vi "Read Sensors v4.vi"(6 "I/O Cluster":T1, 10 "Use Simulation Data?":bool) -> (0 "Vicon Logging Signal":dbl, 3 "Sensors":T19)   [LabVIEW 2018]
uses:
  Sensor Data.ctl
  Target IO Initialized Cluster.ctl
  <vilib>/myRIO/Instrument Drivers/Onboard IO/AI/typedefs/AI Reference.ctl
  <vilib>/myRIO/Common/Instrument Driver Framework/Utilities/typedefs/myRIO Generic Hardware Reference.ctl
  <vilib>/myRIO/Common/Instrument Driver Framework/Utilities/typedefs/Hardware Version Enum.ctl
  <vilib>/myRIO/Common/Instrument Driver Framework/Utilities/typedefs/myRIO v1.0 Reference.ctl
  <vilib>/myRIO/Common/Instrument Driver Framework/Utilities/typedefs/Generic FPGA Reference.ctl
  <vilib>/myRIO/Common/Instrument Driver Framework/myRIO v1.0/AI/typedefs/AI Channels List.ctl
  <vilib>/myRIO/Common/Instrument Driver Framework/myRIO v1.0/AI/typedefs/AI Channels Enum.ctl
  <vilib>/myRIO/Common/Instrument Driver Framework/Utilities/typedefs/Analog Scaling Constants List.ctl
  <vilib>/myRIO/Common/Instrument Driver Framework/Utilities/typedefs/Analog Scaling Constants.ctl
  <vilib>/myRIO/Instrument Drivers/Onboard IO/AO/typedefs/AO Reference.ctl
  <vilib>/myRIO/Common/Instrument Driver Framework/myRIO v1.0/AO/typedefs/AO Channels List.ctl
  <vilib>/myRIO/Common/Instrument Driver Framework/myRIO v1.0/AO/typedefs/AO Channels Enum.ctl
  <vilib>/myRIO/Instrument Drivers/Onboard IO/Encoder/typedefs/Encoder Reference.ctl
  <vilib>/myRIO/Common/Instrument Driver Framework/myRIO v1.0/Encoder/typedefs/Encoder Channels Enum.ctl
  <vilib>/myRIO/Instrument Drivers/Onboard IO/DIO/typedefs/DIO Reference.ctl
  <vilib>/myRIO/Common/Instrument Driver Framework/myRIO v1.0/DIO/typedefs/DIO Channels List.ctl
  <vilib>/myRIO/Common/Instrument Driver Framework/myRIO v1.0/DIO/typedefs/DIO Channels Enum.ctl
  <vilib>/myRIO/Instrument Drivers/Onboard IO/AI/AI.lvlib
  <vilib>/myRIO/Instrument Drivers/Onboard IO/AO/AO.lvlib
  <vilib>/myRIO/Instrument Drivers/Onboard IO/Encoder/Encoder.lvlib
  <vilib>/myRIO/Instrument Drivers/Onboard IO/DIO/DIO.lvlib
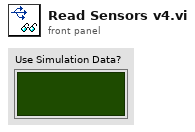
[diagram p1: front panel]
types:
  T1 = typedef "Target IO Initialized Cluster.ctl" = cluster{"AI Ref Out":T2, "AO Ref Out":T11, "Encoder Ref Out":T14, "UART resource name out":refnum<visa-resource-name>, "DIO Ref Out":T16}
  T2 = typedef "AI.lvlib/AI Reference.ctl" = cluster{"myRIO Reference":T3, "AI Channels List":T7, "AI Scaling Constants List":T9}
  T3 = typedef "myRIO Generic Hardware Reference.ctl" = cluster{"myRIO Model":T4, "myRIO Hardware Reference":T5}
  T4 = typedef "Hardware Version Enum.ctl" = enum16{"Unknown", "myRIO-1900", "myRIO-1950", "roboRIO", "NI ELVIS RIO CM", "ELVIS III"}
  T5 = typedef "myRIO v1.0 Reference.ctl" = cluster{"Generic FPGA Reference":T6, "Allow multiple opens":bool}
  T6 = typedef "Generic FPGA Reference.ctl" = refnum<k20>
  T7 = typedef "AI Channels List.ctl" = T8[]
  T8 = typedef "AI Channels Enum.ctl" = enum16{"Not Connected", "AudioIn/Left", "AudioIn/Right", "C/AI0", "C/AI1", "A/AI0", "A/AI1", "A/AI2", "A/AI3", "A/AI4", "A/AI5", "A/AI6", "A/AI7", "B/AI0", "B/AI1", "B/AI2", "B/AI3", "B/AI4", "B/AI5", "B/AI6", "B/AI7", "AI/AI0", "AI/AI1", "AI/AI2", "AI/AI3", "A/AI0 (DIFF)", "A/AI1 (DIFF)", "A/AI2 (DIFF)", "A/AI3 (DIFF)", "B/AI0 (DIFF)", "B/AI1 (DIFF)", "B/AI2 (DIFF)", "B/AI3 (DIFF)"}
  T9 = typedef "Analog Scaling Constants List.ctl" = T10[]
  T10 = typedef "Analog Scaling Constants.ctl" = cluster{"LSB Weight (Volts)":dbl, "Offset (Volts)":dbl, "Signed?":bool}
  T11 = typedef "AO.lvlib/AO Reference.ctl" = cluster{"myRIO Reference":T3, "AO Channel List":T12, "AO Scaling Constant List":T9}
  T12 = typedef "AO Channels List.ctl" = T13[]
  T13 = typedef "AO Channels Enum.ctl" = enum16{"Not Connected", "AudioOut/Left", "AudioOut/Right", "C/AO0", "C/AO1", "A/AO0", "A/AO1", "B/AO0", "B/AO1"}
  T14 = typedef "Encoder.lvlib/Encoder Reference.ctl" = cluster{"myRIO Reference":T3, "Encoder Channels Enum":T15}
  T15 = typedef "Encoder Channels Enum.ctl" = enum16{"Not Connected", "C/ENC0", "C/ENC1", "A/ENC", "A/ENC0", "A/ENC1", "A/ENC2", "A/ENC3", "A/ENC4", "A/ENC5", "A/ENC6", "A/ENC7", "A/ENC8", "A/ENC9", "B/ENC", "B/ENC0", "B/ENC1", "B/ENC2", "B/ENC3", "B/ENC4", "B/ENC5", "B/ENC6", "B/ENC7", "B/ENC8", "B/ENC9", "DIO/ENC0", "DIO/ENC1", "DIO/ENC2", "DIO/ENC3", "DIO/ENC4"}
  T16 = typedef "DIO.lvlib/DIO Reference.ctl" = cluster{"myRIO Reference":T3, "DIO Channels List":T17}
  T17 = typedef "DIO Channels List.ctl" = T18[]
  T18 = typedef "DIO Channels Enum.ctl" = enum16{"Not Connected", "C/DIO0", "C/DIO1", "C/DIO2", "C/DIO3", "C/DIO4", "C/DIO5", "C/DIO6", "C/DIO7", "A/DIO0", "A/DIO1", "A/DIO2", "A/DIO3", "A/DIO4", "A/DIO5", "A/DIO6", "A/DIO7", "A/DIO8", "A/DIO9", "A/DIO10", "A/DIO11", "A/DIO12", "A/DIO13", "A/DIO14", "A/DIO15", "A/DIO16", "A/DIO17", "A/DIO18", "A/DIO19", "B/DIO0", "B/DIO1", "B/DIO2", "B/DIO3", "B/DIO4", "B/DIO5", "B/DIO6", "B/DIO7", "B/DIO8", "B/DIO9", "B/DIO10", "B/DIO11", "B/DIO12", "B/DIO13", "B/DIO14", "B/DIO15", "B/DIO16", "B/DIO17", "B/DIO18", "B/DIO19", "LED0", "LED1", "LED2", "LED3", "Button0", "DIO/DIO0", "DIO/DIO1", "DIO/DIO2", "DIO/DIO3", "DIO/DIO4", "DIO/DIO5", "DIO/DIO6", "DIO/DIO7", "DIO/DIO8", "DIO/DIO9", "SPI/CS0", "SPI/CS1", "SPI/CS2", "SPI/CS3", "LED RADIO (Green)", "LED RADIO (Red)", "LED COMM (Green)", "LED COMM (Red)", "LED MODE (Green)", "LED MODE (Red)"}
  T19 = typedef "Sensor Data.ctl" = cluster{"Motor Current":dbl, "Motor Velocity":dbl, "Ankle Encoder Angle":dbl, "GRF L":dbl, "GRF R":dbl, "Index pulse?":bool, "Roll":dbl, "Pitch":dbl, "Yaw":dbl, "Thigh Angle":dbl}
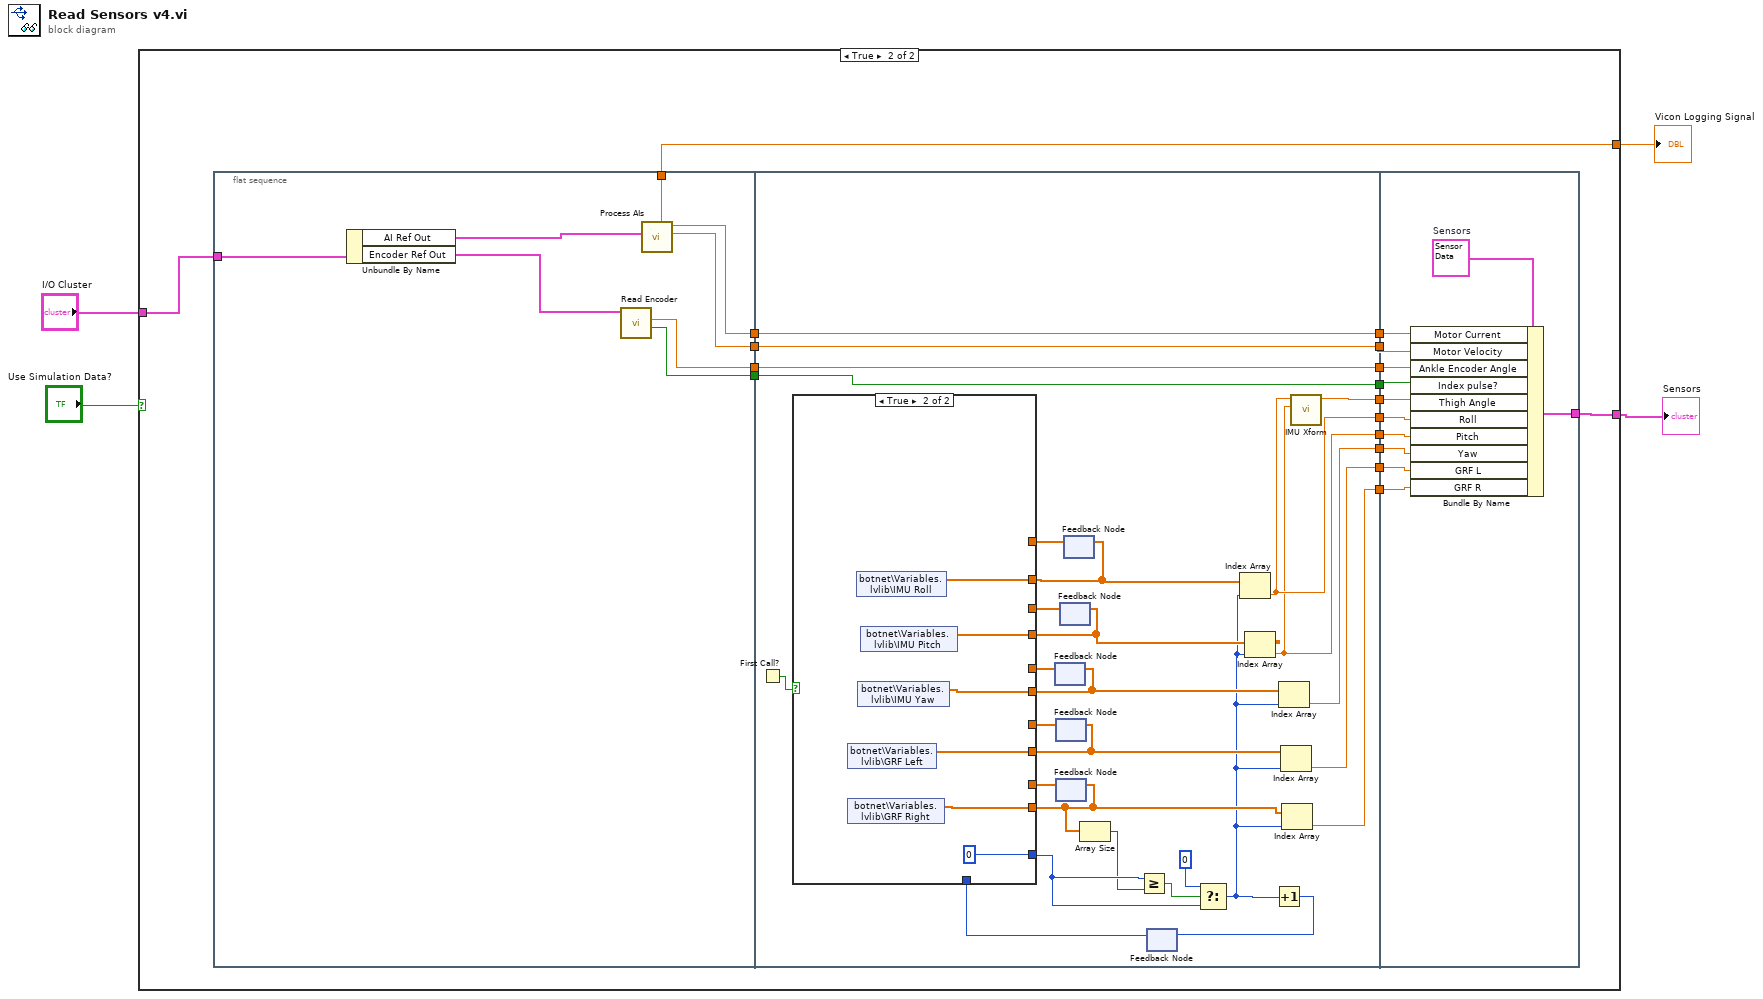
[diagram p0: block diagram]
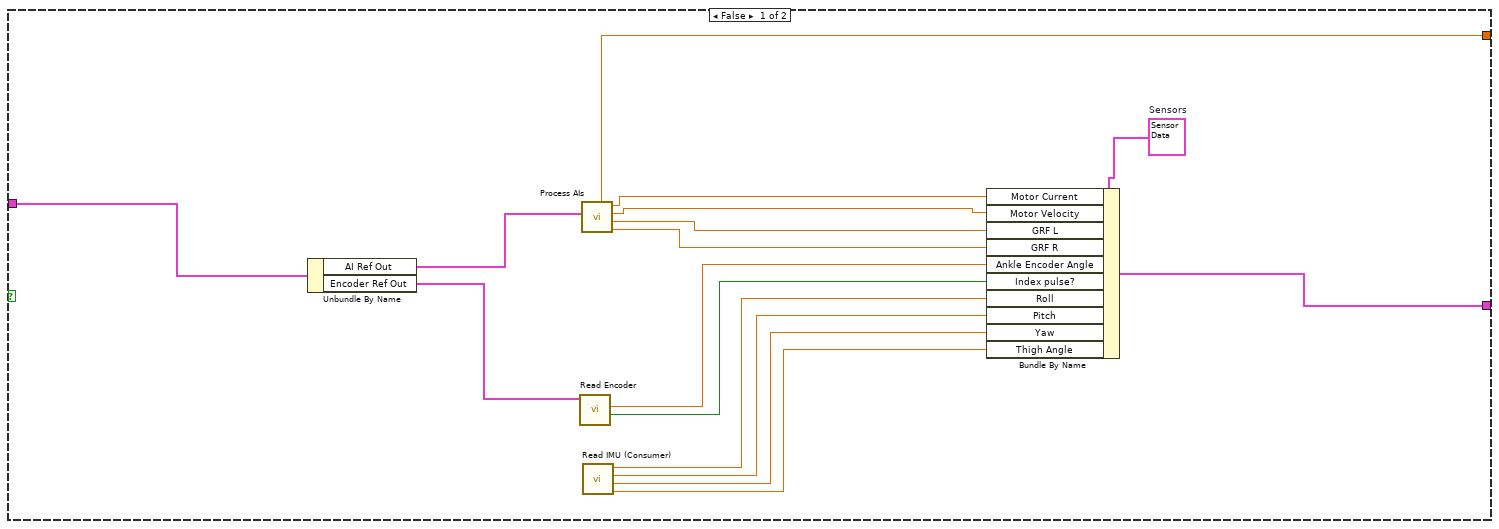
[diagram p2: hidden frame]
diagram:
  n1 = case shown="True" "Use Simulation Data?" {
    tunnel: [w19 w37] -> w4
    tunnel: "I/O Cluster" -> [w6 w23]
    tunnel: [w5 w22] -> w1
    frame False {
      w20 = T19 {"Motor Current"=0.0, "Motor Velocity"=0.0, "Ankle Encoder Angle"=0.0, "GRF L"=0.0, "GRF R"=0.0, "Index pulse?"=FALSE, "Roll"=0.0, "Pitch"=0.0, "Yaw"=0.0, "Thigh Angle"=0.0}  # Sensors
      n2 = Unbundle By Name(w6) -> ("AI Ref Out"=w11:T2, "Encoder Ref Out"=w18:T14)
      n3 = call "Read Encoder.vi"("Encoder Ref In"=w18) -> ("Has Index Pulse Occured \nthis Run?"=w16:bool, "Angular Encoder Abs.\nDisplacement (rad)"=w17:dbl)  [unwired: 8 in, 1 out]
      n4 = call "Process AIs.vi"("AI Ref In"=w11) -> ("GRF R"=w7:dbl, "GRF L"=w8:dbl, "Motor Velocity"=w9:dbl, "Actual Motor Current"=w10:dbl, "Vicon Trigger Signal"=w5:dbl)  [unwired: 5 in, 1 out]
      n5 = call "Read IMU (Consumer).vi"() -> ("Thigh Angle [rad]"=w12:dbl, "Yaw Angle [rad]"=w13:dbl, "Pitch Angle [rad]"=w14:dbl, "Roll Angle [rad]"=w15:dbl)  [unwired: 8 in]
      n6 = Bundle By Name(cluster=w20, "Motor Current"=w10, "Motor Velocity"=w9, "GRF L"=w8, "GRF R"=w7, "Ankle Encoder Angle"=w17, "Index pulse?"=w16, "Roll"=w15, "Pitch"=w14, "Yaw"=w13, "Thigh Angle"=w12) -> (w19:T19)
    }
    frame True {
      n7 = flat-sequence {
        tunnel: [w44] -> w36
        tunnel: [w43] -> w34
        tunnel: [w41] -> w32
        tunnel: [w40] -> w30
        tunnel: w23 -> [w39]
        tunnel: [w38] -> w22
        tunnel: w36 -> [w73]
        tunnel: [w73] -> w35
        tunnel: w34 -> [w72]
        tunnel: [w72] -> w33
        tunnel: w32 -> [w71]
        tunnel: [w71] -> w31
        tunnel: w30 -> [w70]
        tunnel: [w70] -> w29
        tunnel: [w47] -> w28
        tunnel: [w46] -> w27
        tunnel: [w51] -> w26
        tunnel: [w50] -> w25
        tunnel: [w49] -> w24
        tunnel: [w48] -> w21
        tunnel: w35 -> [w95]
        tunnel: w33 -> [w94]
        tunnel: w31 -> [w97]
        tunnel: w29 -> [w96]
        tunnel: [w93] -> w37
        tunnel: w28 -> [w91]
        tunnel: w27 -> [w90]
        tunnel: w26 -> [w89]
        tunnel: w25 -> [w88]
        tunnel: w24 -> [w87]
        tunnel: w21 -> [w86]
        frame #0 {
          n8 = Unbundle By Name(w39) -> ("AI Ref Out"=w42:T2, "Encoder Ref Out"=w45:T14)
          n9 = call "Read Encoder.vi"("Encoder Ref In"=w45) -> ("Has Index Pulse Occured \nthis Run?"=w43:bool, "Angular Encoder Abs.\nDisplacement (rad)"=w44:dbl)  [unwired: 8 in, 1 out]
          n10 = call "Process AIs.vi"("AI Ref In"=w42) -> ("Motor Velocity"=w40:dbl, "Actual Motor Current"=w41:dbl, "Vicon Trigger Signal"=w38:dbl)  [unwired: 5 in, 3 out]
        }
        frame #1 {
          n11 = First Call?() -> (First Call?: T/F=w52:bool)
          n12 = feedback #1() -> (w67:dbl[])  [unwired: 1 in]
          n13 = feedback #2() -> (w66:dbl[])  [unwired: 1 in]
          n14 = feedback #3() -> (w65:dbl[])  [unwired: 1 in]
          n15 = feedback #4() -> (w68:dbl[])  [unwired: 1 in]
          n16 = feedback #5() -> (w69:dbl[])  [unwired: 1 in]
          n17 = feedback #6() -> (w63:i32)  [unwired: 1 in]
          n18 = case shown="True" w52 {
            tunnel: [w79 w85] -> w58
            tunnel: w69 -> [w79 _]
            tunnel: [w78 w84] -> w57
            tunnel: [w77 w83] -> w56
            tunnel: [w76 w82] -> w55
            tunnel: [w75 w80] -> w54
            tunnel: w68 -> [w78 _]
            tunnel: w67 -> [w77 _]
            tunnel: w66 -> [w76 _]
            tunnel: w65 -> [w75 _]
            tunnel: [w74 0] -> w60
            tunnel: w63 -> [w74 _]
            frame False {
            }
            frame True {
              n19 = shared-variable "botnet\\Variables.lvlib\\GRF Left"() -> (w82:dbl[])  [unwired: 1 in, 1 out]
              n20 = shared-variable "botnet\\Variables.lvlib\\GRF Right"() -> (w80:dbl[])  [unwired: 1 in, 1 out]
              n21 = shared-variable "botnet\\Variables.lvlib\\IMU Roll"() -> (w85:dbl[])  [unwired: 1 in, 1 out]
              n22 = shared-variable "botnet\\Variables.lvlib\\IMU Yaw"() -> (w83:dbl[])  [unwired: 1 in, 1 out]
              n23 = shared-variable "botnet\\Variables.lvlib\\IMU Pitch"() -> (w84:dbl[])  [unwired: 1 in, 1 out]
            }
          }
          n24 = feedback-in #1(w56) -> ()
          n25 = feedback-in #2(w55) -> ()
          n26 = feedback-in #3(w54) -> ()
          n27 = feedback-in #4(w57) -> ()
          n28 = feedback-in #5(w58) -> ()
          n29 = Array Size(array=w54) -> (size(s)=w59:i32)
          n30 = Greater Or Equal?(x=w60, y=w59) -> (x >= y?=w61:bool)
          n31 = Select(t=0, s=w61, f=w60) -> (s? t:f=w53:i32)
          n32 = Index Array(array=w58, index=w53) -> (element=w47:dbl)
          n33 = Index Array(array=w57, index=w53) -> (element=w46:dbl)
          n34 = Increment(x=w53) -> (x+1=w64:i32)
          n35 = feedback-in #6(w64) -> ()
          n36 = Index Array(array=w56, index=w53) -> (element=w51:dbl)
          n37 = Index Array(array=w55, index=w53) -> (element=w50:dbl)
          n38 = Index Array(array=w54, index=w53) -> (element=w49:dbl)
          n39 = call "IMU Xform.vi"("Pitch"=w46, "Roll"=w47) -> ("Thigh Angle"=w48:dbl)  [unwired: 9 in]
        }
        frame #2 {
          w92 = T19 {"Motor Current"=0.0, "Motor Velocity"=0.0, "Ankle Encoder Angle"=0.0, "GRF L"=0.0, "GRF R"=0.0, "Index pulse?"=FALSE, "Roll"=0.0, "Pitch"=0.0, "Yaw"=0.0, "Thigh Angle"=0.0}  # Sensors
          n40 = Bundle By Name(cluster=w92, "Motor Current"=w97, "Motor Velocity"=w96, "Ankle Encoder Angle"=w95, "Index pulse?"=w94, "Thigh Angle"=w86, "Roll"=w91, "Pitch"=w90, "Yaw"=w89, "GRF L"=w88, "GRF R"=w87) -> (w93:T19)
        }
      }
    }
  }
  "Sensors" <- w4
  "Vicon Logging Signal" <- w1
